vi "PSVCH_Formula Check.vi"(8 "Error In (no error)":errorcluster, 10 "VarList":T6, 11 "Formula":string) -> (0 "Error Out":errorcluster, 1 "Formula Node 2":T1, 2 "source":string, 3 "code":i32, 5 "VarList":T5)   [LabVIEW 2016]
uses:
  Ctrls/PSVCH_VarList.ctl
  ShareLib/Formula/Ctrls/PSFormula_FOR_Formula Node.ctl
  ShareLib/Formula/Ctrls/PSFormula_FOR_Formula Step.ctl
  ShareLib/Formula/Ctrls/PSFormula_FOR_Formula Para.ctl
  ShareLib/Formula/Ctrls/PSFormula_FOR_Formula MidVar Data.ctl
  Ctrls/PSVCH_Formula MidVar Data.ctl
  <vilib>/Pansino Software/ToolkitLib/VARIANT Tool/Ctrls/PSVARIANT_Variant Para.ctl
  <vilib>/Pansino Software/ToolkitLib/VARIANT Tool/Ctrls/PSVARIANT_Data Type.ctl
panel:
  # "Data Out"
  # "Data In"
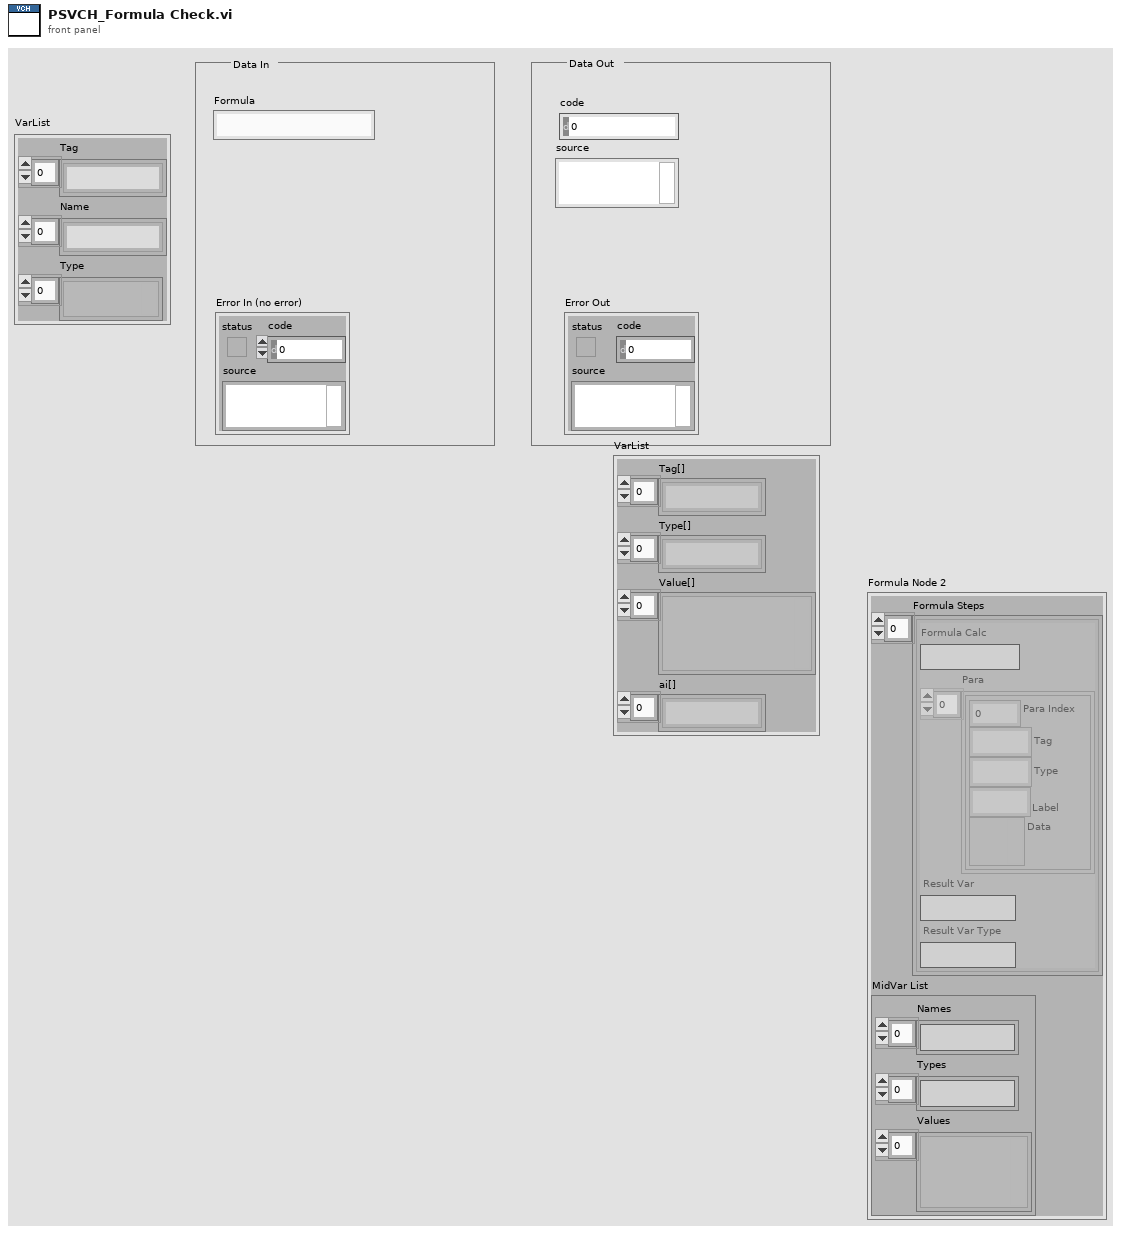
[diagram p1: front panel]
types:
  T1 = typedef "PSFormula_FOR_Formula Node.ctl" = cluster{"Formula Steps":T2[], "MidVar List":T4}
  T2 = typedef "PSFormula_FOR_Formula Step.ctl" = cluster{"Formula Calc":string, "Para":T3[], "Result Var":string, "Result Var Type":string}
  T3 = typedef "PSFormula_FOR_Formula Para.ctl" = cluster{"Para Index":i32, "Tag":string, "Type":string, "Label":string, "Data":variant}
  T4 = typedef "PSFormula_FOR_Formula MidVar Data.ctl" = cluster{"Names":string[], "Types":string[], "Values":variant[]}
  T5 = typedef "PSVCH_VarList.ctl" = cluster{"Tag[]":string[], "Type[]":string[], "Value[]":variant[], "ai[]":string[]}
  T6 = cluster{"Tag":string[], "Name":string[], "Type":variant[]}
  T7 = typedef "PSVCH_Formula MidVar Data.ctl" = cluster{"Names":string[], "Types":string[], "Values":variant[]}
  T8 = typedef "PSVARIANT_Variant Para.ctl" = cluster{"Label":string, "Type Data":T9[], "Type String":string, "Array Dimension":i32, "Variant":variant}
  T9 = typedef "PSVARIANT_Data Type.ctl" = u8
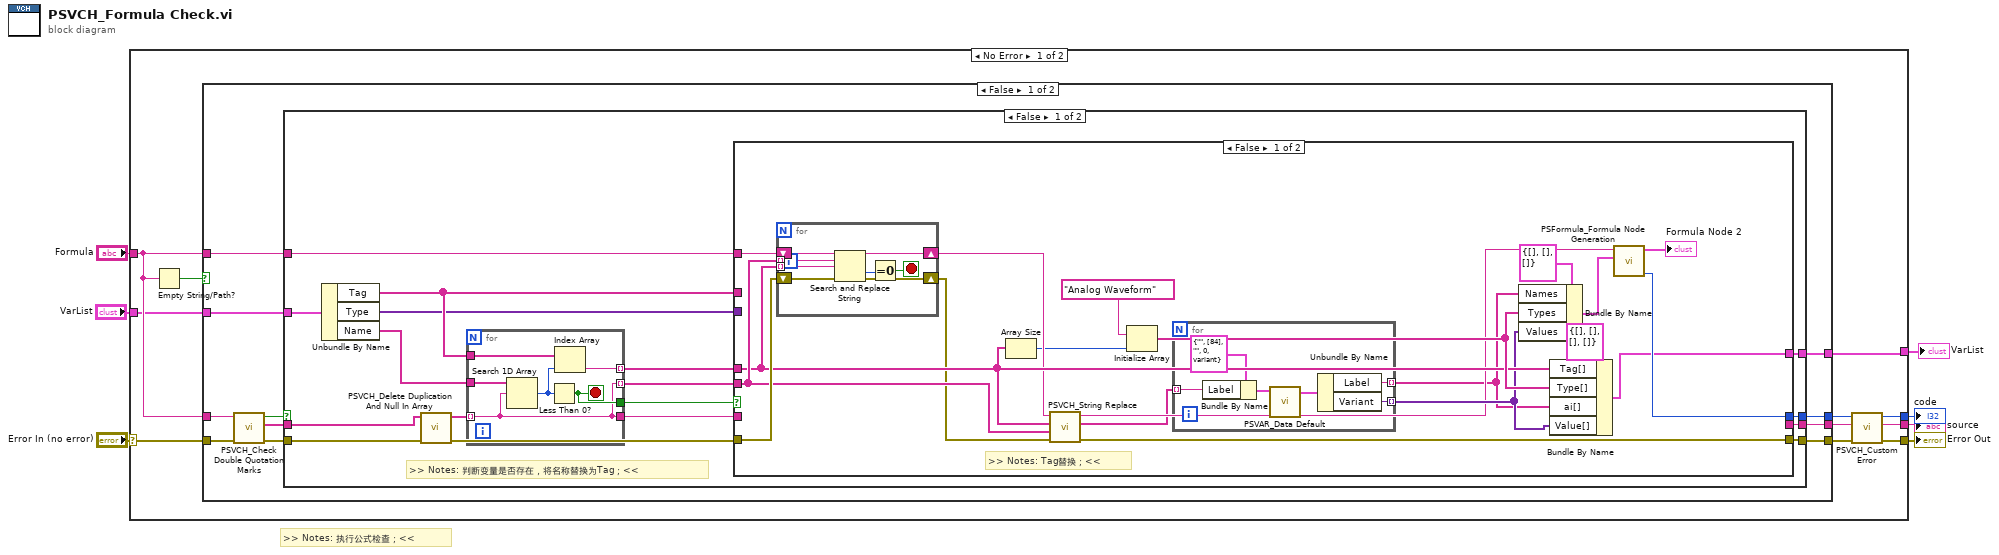
[diagram p0: block diagram]
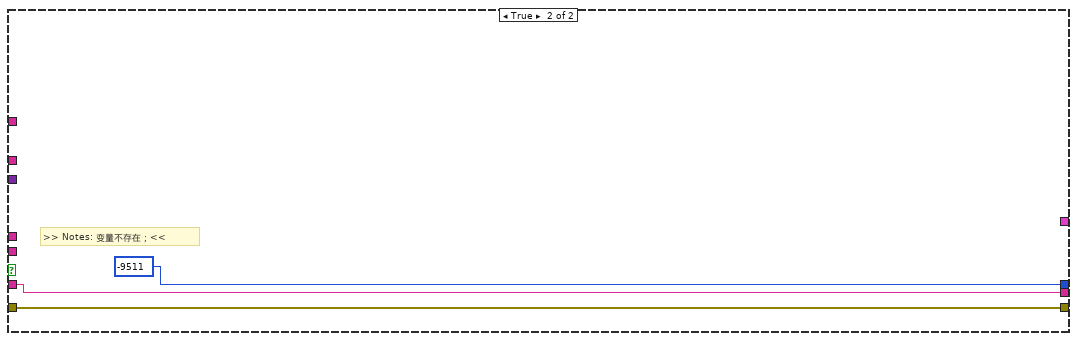
[diagram p2: hidden frame]
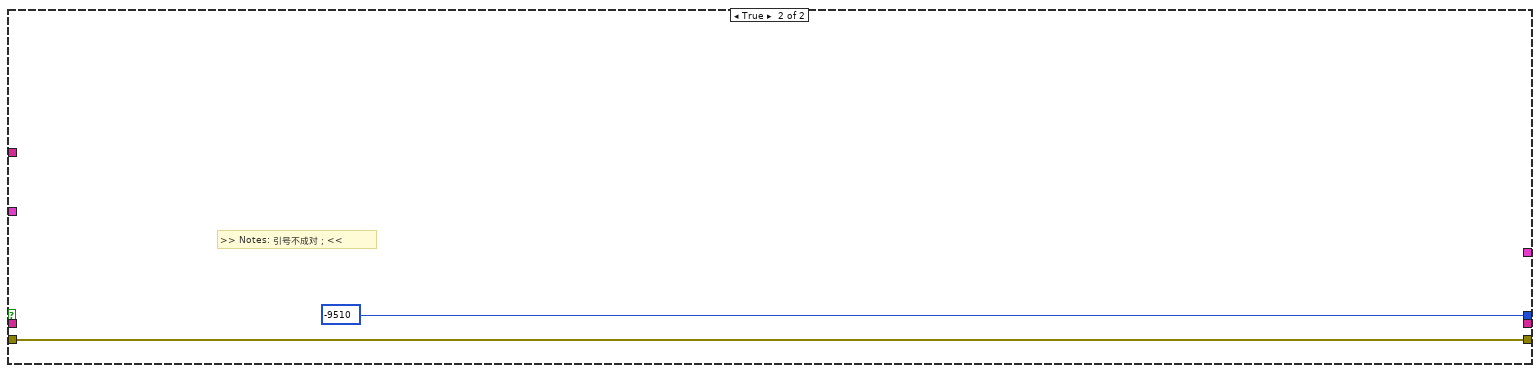
[diagram p3: hidden frame]
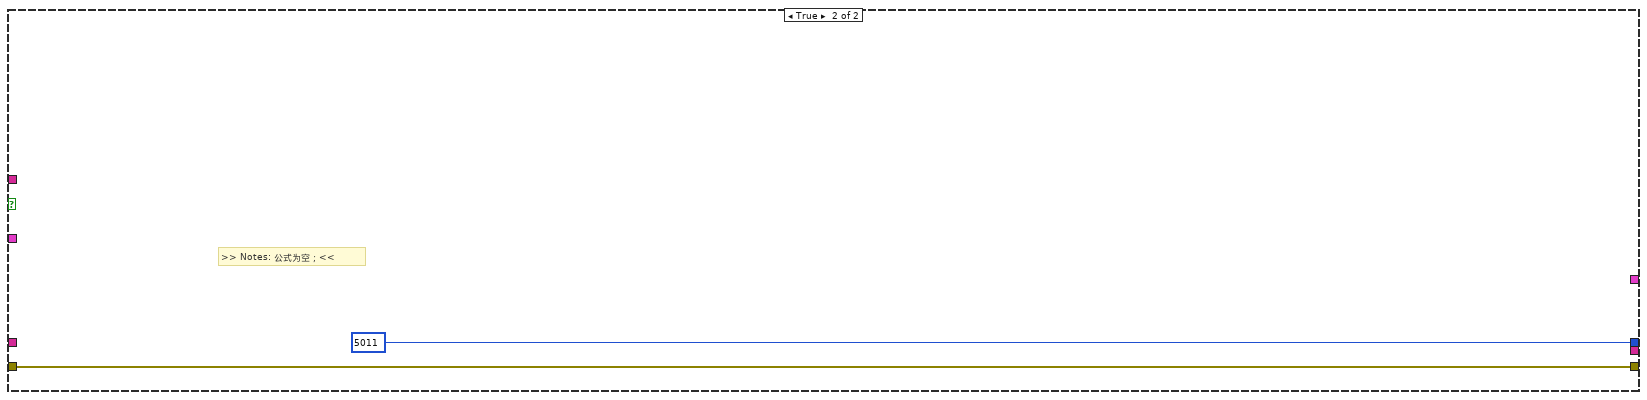
[diagram p4: hidden frame]
diagram:
  # ">> Notes: 执行公式检查；<<"
  n1 = case shown="No Error" "Error In (no error)" {
    selector: "Error In (no error)" -> [w17 w94]
    tunnel: [w14 w94] -> w5
    tunnel: "Formula" -> [w16 _]
    tunnel: [w13 _] -> w4
    tunnel: [w12 _] -> w3
    tunnel: "VarList" -> [w9 _]
    tunnel: [w8 _] -> w1
    frame No Error {
      n2 = Empty String/Path?(string/path=w16) -> (empty?=w18:bool)
      n3 = case shown="False" w18 {
        tunnel: w17 -> [w27 w92]
        tunnel: [w29 w92] -> w15
        tunnel: w16 -> [w23 _]
        tunnel: w16 -> [w28 _]
        tunnel: [w22 5011 ("Custom Code")] -> w11
        tunnel: [w21 _] -> w10
        tunnel: w9 -> [w20 _]
        tunnel: [w19 _] -> w8
        frame False {
          n4 = call "PSVCH_Check Double Quotation Marks.vi"("Error In (no error)"=w27, "String"=w23) -> ("Error Out"=w26:errorcluster, "\"Tag\"[]"=w25:string[], "Error?"=w24:bool)  [unwired: 7 in]
          n5 = case shown="False" w24 {
            tunnel: w26 -> [w38 w91]
            tunnel: [w43 w91] -> w29
            tunnel: w25 -> [w46 _]
            tunnel: w28 -> [w39 _]
            tunnel: [w36 -9510 ("Error Code")] -> w22
            tunnel: [w35 _] -> w21
            tunnel: w20 -> [w34 _]
            tunnel: [w30 _] -> w19
            frame False {
              # ">> Notes: 判断变量是否存在，将名称替换为Tag；<<"
              n6 = Unbundle By Name(w34) -> ("Tag"=w33:string[], "Type"=w32:variant[], "Name"=w31:string[])
              n7 = call "PSVCH_Delete Duplication And Null In Array.vi"("Error In (no error)"=w38, "ArrayIn"=w46) -> ("Error Out"=w37:errorcluster, "ArrayOut"=w45:string[])  [unwired: 8 in]
              n8 = for {
                tunnel: w45 -> [w84] mode=indexing
                tunnel: w31 -> [w89]
                tunnel: [w84] -> w42
                tunnel: [w88] -> w44
                tunnel: w33 -> [w86]
                tunnel: [w85] -> w41 mode=indexing
                tunnel: [w84] -> w40 mode=indexing
                stop <- w88 stop-if-true
                n9 = Search 1D Array(1D array=w89, element=w84) -> (index of element=w87:i32)  [unwired: 1 in]
                n10 = Less Than 0?(x=w87) -> (x < 0?=w88:bool)
                n11 = Index Array(array=w86, index=w87) -> (element=w85:string)
              }
              n12 = case shown="False" w44 {
                tunnel: w37 -> [w58 w83]
                tunnel: [w66 w83] -> w43
                tunnel: w42 -> [_ w81]
                tunnel: w41 -> [w56 _]
                tunnel: w40 -> [w57 _]
                tunnel: w39 -> [w54 _]
                tunnel: w33 -> [_ _]
                tunnel: w32 -> [_ _]
                tunnel: [w63 -9511 ("Error Code")] -> w36
                tunnel: [_ w81] -> w35
                tunnel: [w59 _] -> w30
                frame False {
                  # ">> Notes: Tag替换；<<"
                  n13 = for {
                    shift-right: [w76] -> w53
                    shift-left: w54 -> [w80]
                    tunnel: w57 -> [w78] mode=indexing
                    tunnel: w56 -> [w77] mode=indexing
                    shift-right: [w73] -> w55
                    shift-left: w58 -> [w79]
                    stop <- w74 stop-if-true
                    n14 = Search and Replace String(input string=w80, search string=w78, replace string=w77, error in=w79) -> (result string=w76:string, offset past replacement=w75:i32, error out=w73:errorcluster)  [unwired: 4 in, 1 out]
                    n15 = Equal To 0?(x=w75) -> (x = 0?=w74:bool)
                  }
                  n16 = Array Size(array=w56) -> (size(s)=w52:i32)
                  n17 = call "PSVCH_String Replace.vi"("Error In (no error)"=w55, "ai[] In"=w57, "Tag[] In"=w56, "String In"=w53) -> ("Error Out"=w66:errorcluster, "ai[] Out"=w49:string[], "String Out"=w50:string)  [unwired: 4 in, 1 out]
                  n18 = Initialize Array("Analog Waveform", w52) -> (w60:string[])
                  n19 = for {
                    tunnel: [w69] -> w51 mode=indexing
                    tunnel: [w68] -> w48 mode=indexing
                    tunnel: w49 -> [w67] mode=indexing
                    n20 = Bundle By Name(cluster=T8 {"Label"="", "Type Data"=[84], "Type String"="", "Array Dimension"=0, "Variant"=variant} ("Data In"), "Label"=w67) -> (w71:T8)
                    n21 = call <vilib>:"PSVAR_Data Default.vi"("Data In"=w71) -> ("Data Default"=w70:T8)  [unwired: 9 in, 1 out]
                    n22 = Unbundle By Name(w70) -> ("Label"=w68:string, "Variant"=w69:variant)
                  }
                  n23 = Bundle By Name(cluster=T7 {"Names"=[], "Types"=[], "Values"=[]} ("Var List"), "Names"=w48, "Types"=w60, "Values"=w51) -> (w64:T7)
                  n24 = Bundle By Name(cluster=T5 {"Tag[]"=[], "Type[]"=[], "Value[]"=[], "ai[]"=[]} ("输出簇"), "Tag[]"=w56, "Type[]"=w60, "ai[]"=w48, "Value[]"=w51) -> (w59:T5)
                  n25 = call "PSFormula_Formula Node Generation.vi"("Var List"=w64, "Fomula"=w50) -> ("Error Code"=w63:i32, "Formula Node"=→"Formula Node 2":T1)  [unwired: 8 in]
                }
                frame True {
                  # ">> Notes: 变量不存在；<<"
                }
              }
            }
            frame True {
              # ">> Notes: 引号不成对；<<"
            }
          }
        }
        frame True {
          # ">> Notes: 公式为空；<<"
        }
      }
      n26 = call "PSVCH_Custom Error.vi"("error in (no error)"=w15, "Source"=w10, "Custom Code"=w11) -> ("error out"=w14:errorcluster, "Explanation"=w12:string, "Custom Code"=w13:i32)  [unwired: 6 in]
    }
    frame Error {
    }
  }
  "Error Out" <- w5
  "code" <- w4
  "source" <- w3
  "VarList" <- w1
